vi "DP-Artifact Rejection V2.vi"(5 "Magnitude (Vrms)":dbl[](array[numeric]), 7 "df (kHz)":dbl, 8 "DP Freqs":T2, 9 "Mic gain (dB)":dbl, 10 "Probe Tube Sensitivity":cluster{"Frequency":dbl[], "Mag":dbl[]}, 11 "Reject Ref":T1) -> (3 "Reject?":bool)   [LabVIEW 2020]
uses:
  Typedefs/DP-Freqs.ctl
  Typedefs/DP-Rejection Settings Refnum.ctl
  Typedefs/DP-Rejection Settings.ctl
  Utility VIs/Math VIs/Linear to dB (scalar).vi
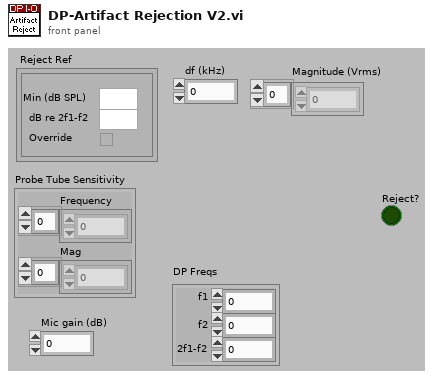
[diagram p1: front panel]
types:
  T1 = typedef "DP-Rejection Settings Refnum.ctl" = refnum<vi>
  T2 = typedef "DP-Freqs.ctl" = cluster{"f1":dbl, "f2":dbl, "2f1-f2":dbl}
  T3 = typedef "DP-Rejection Settings.ctl" = cluster{"Override":bool, "dB re 2f1-f2":dbl, "Min (dB SPL)":dbl}
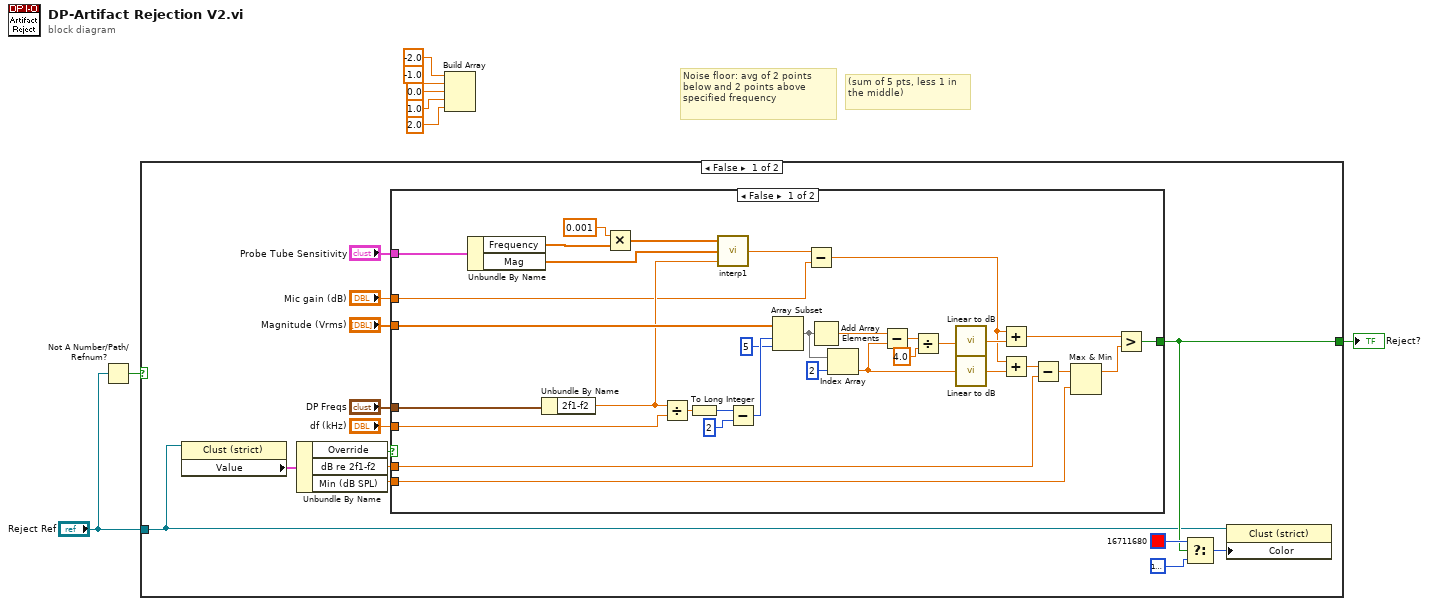
[diagram p0: block diagram]
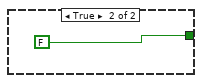
[diagram p2: hidden frame]
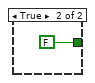
[diagram p3: hidden frame]
diagram:
  # "(sum of 5 pts, less 1 in the middle)"
  # "Noise floor: avg of 2 points\nbelow and 2 points above specified frequency"
  n1 = Not A Number/Path/Refnum?(number/path/refnum="Reject Ref") -> (NaN/Path/Refnum?=w2:bool)
  n2 = case shown="False" w2 {
    tunnel: [w13 FALSE] -> w8
    tunnel: "Reject Ref" -> [w12 _]
    frame False {
      n3 = property class="Clust (strict)"(reference=w12) -> ("Value"=w18:T3)  [unwired: 1 in, 2 out]
      n4 = Unbundle By Name(w18) -> ("Override"=w20:bool, "dB re 2f1-f2"=w19:dbl, "Min (dB SPL)"=w17:dbl)
      n5 = case shown="False" w20 {
        tunnel: "DP Freqs" -> [w54 _]
        tunnel: "Magnitude (Vrms)" -> [w41 _]
        tunnel: [w46 FALSE] -> w13
        tunnel: w19 -> [w30 _]
        tunnel: w17 -> [w28 _]
        tunnel: "df (kHz)" -> [w25 _]
        tunnel: "Mic gain (dB)" -> [w24 _]
        tunnel: "Probe Tube Sensitivity" -> [w23 _]
        frame False {
          n6 = Unbundle By Name(w23) -> ("Frequency"=w45:dbl[], "Mag"=w42:dbl[])
          n7 = Unbundle By Name(w54) -> ("2f1-f2"=w38:dbl)
          n8 = Multiply(x=0.001, y=w45) -> (x*y=w43:dbl[])
          n9 = Divide(x=w38, y=w25) -> (x/y=w55:dbl)
          n10 = To Long Integer(number=w55) -> (32bit integer=w53:i32)
          n11 = call "interp1.vi"("X"=w43, "Y"=w42, "U"=w38) -> ("V"=w35:dbl)  [unwired: 2 in]
          n12 = Subtract(x=w53, y=2) -> (x-y=w51:i32)
          n13 = Array Subset(array=w41, index=w51, length=5) -> (w40:dbl[])
          n14 = Subtract(x=w35, y=w24) -> (x-y=w33:dbl)
          n15 = Add Array Elements(numeric array=w40) -> (sum=w47:dbl)
          n16 = Index Array(array=w40, index=2) -> (element=w36:dbl)
          n17 = Subtract(x=w47, y=w36) -> (x-y=w49:dbl)
          n18 = Divide(x=w49, y=4.0) -> (x/y=w37:dbl)
          n19 = call-poly "Linear to dB.vi"("Linear"=w37) -> ("dB"=w34:dbl)
          n20 = call-poly "Linear to dB.vi"("Linear"=w36) -> ("dB"=w32:dbl)
          n21 = Add(x=w33, y=w34) -> (x+y=w26:dbl)
          n22 = Add(x=w33, y=w32) -> (x+y=w31:dbl)
          n23 = Subtract(x=w31, y=w30) -> (x-y=w29:dbl)
          n24 = Max & Min(x=w29, y=w28) -> (max(x,y)=w27:dbl)  [unwired: 1 out]
          n25 = Greater?(x=w26, y=w27) -> (0:w46:bool)
        }
        frame True {
        }
      }
      n26 = Select(t=u32 16711680, s=w13, f=u32 16777238) -> (s? t:f=w14:u32)
      n27 = property class="Clust (strict)"(reference=w12, "Color"=w14) -> ()  [unwired: 1 in, 2 out]
    }
    frame True {
    }
  }
  "Reject?" <- w8
  n28 = Build Array(-2.0, -1.0, 0.0, 1.0, 2.0) -> ()  [unwired: 1 out]
